vi "Sum of 20 Natural Numbers.vi"() -> ()   [LabVIEW 2018]
panel:
  out "Result":dbl
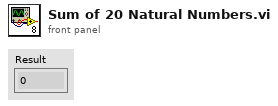
[diagram p1: front panel]
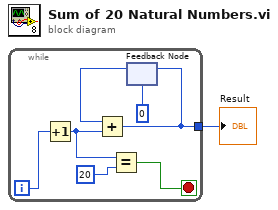
[diagram p0: block diagram]
diagram:
  n1 = while {
    tunnel: [w8] -> w1
    i -> [w3]
    stop <- w5 stop-if-true
    n2 = Increment(x=w3) -> (x+1=w2:i32)
    n3 = Equal?(x=w2, y=20) -> (x = y?=w5:bool)
    n4 = feedback #1(0) -> (w7:i32)
    n5 = Add(x=w7, y=w2) -> (x+y=w8:i32)
    n6 = feedback-in #1(w8) -> ()
  }
  "Result" <- w1
